vi "tkrsa6100 Status Regs.vi"(0 "VISA Resource Name":refnum<visa-resource-name>, 5 "Set/Read\nStatus Register (SET)":enum16{"SET", "READ"}(ring), 7 "Register (PRESET)":T1(ring), 9 "Register # (0)":i32 max=32767 step=1, 11 "error in (no error)":errorcluster {"code" format="%#.0f"}) -> (4 "dup VISA Resource Name":refnum<visa-resource-name>, 6 "Register #\nResponse String":string, 8 "Register Bits Array":bool[](array[boolean]), 10 "Register #":i32, 15 "error out":errorcluster {"code" format="%#.0f"})   [LabVIEW 2020, in "Library Instrument & Equipement.lvlib" / "Library Spectrum Analyser.lvlib"]
doc: "Prerequisites for use:\n\nNone. This VI is valid in all measurement views.\n\nThis VI sets or reads the current instrument status registers. To use the VI pass either SET or READ to enumerated control Set/Read Acquisition Setting(SET), pass the input register to be written or read to enumerated control Register(PRESET), and if writing a register, pass the number to numeric control Register # (0). Functions that are write-only are followed by (SET), functions that are read-only are followed by (READ). \n\nFirst error in (no error) is checked by tkrsa6100 Write/Read WError Query.vi for any pending errors.\n\nIf error in status is ERROR:\n\nerror in (no error) and VISA Resource Name are passed straight through to error out and dup VISA Resource Name of the tkrsa6100 Write/Read WError Query.vi and returned to the calling function. No commands are processed.\n\nIf error in status is NO ERROR:\n\nThe register settings are set or read per the values passed to controls Register(PRESET) and Register #(0).\n\nIf SET is passed the following registers can be written per the value passed to numeric control Register # (0): \n\nPRESET (SET). This presets the registers to their default settings. No other parameters are necessary to be passed.\n\nThe following are the registers that can be written:\n\nOPERATION:ENABLE\nOPERATION:PTRANSITION\nOPERATION:NTRANSITION\nQUESTIONABLE:ENABLE\nQUESTIONABLE:PTRANSITION\nQUESTIONABLE:NTRANSITION\nQUESTIONABLE:FREQUENCY:ENABLE\nQUESTIONABLE: FREQUENCY:PTRANSITION\nQUESTIONABLE: FREQUENCY:NTRANSITION\n*QUESTIONABLE:INTEGRITY:ENABLE\n*QUESTIONABLE: INTEGRITY:PTRANSITION\n*QUESTIONABLE: INTEGRITY:NTRANSITION\nQUESTIONABLE:CALIBRATION:ENABLE\nQUESTIONABLE: CALIBRATION:PTRANSITION\nQUESTIONABLE: CALIBRATION:NTRANSITION\n*QUESTIONABLE:POWER:ENABLE\n*QUESTIONABLE: POWER:PTRANSITION\n*QUESTIONABLE: POWER:NTRANSITION\n*QUESTIONABLE:TEMPERATURE:ENABLE\n*QUESTIONABLE: TEMPERATURE:PTRANSITION\n*QUESTIONABLE: TEMPERATURE:NTRANSITION\n\n*These registers currently have no bits assigned in them but are included for completeness.\n\nValues 0 to 32767 can be written to the registers\n.\nWrite a 1 to the bit of interest in the ENABLE registers to enable them.\n\nIf a 1 is written to the bit of interest in the PTRANSITION register the bit will be set in the EVENT register if a low to high transition is detected.\n\nIf a 1 is written to the bit of interest in the NTRANSITION register the bit will be set in the EVENT register if a high to low transition is detected.\n\nIf a 1 is written to the bit of interest in both the PTRANSITION and NTRANSITION registers the bit will be set in the EVENT register if any transition is detected.\n\nRefer to Section 3 (Status and Events) of the Programmer's Manual for assigned register bits and further information.\n\nAfter the correct command string is selected it is passed to tkrsa6100 Write/Read wError Query.vi.\n\nIf READ is passed the following registers can be read.\n\nOPERATION:CONDITION\nOPERATION:ENABLE\nOPERATION:EVENT\nOPERATION:PTRANSITION\nOPERATION:NTRANSITION\nQUESTIONABLE:CONDITION\nQUESTIONABLE:ENABLE\nQUESTIONABLE:EVENT\nQUESTIONABLE:PTRANSITION\nQUESTIONABLE:NTRANSITION\nQUESTIONABLE: FREQUENCY:CONDITION\nQUESTIONABLE:FREQUENCY:ENABLE\nQUESTIONABLE: FREQUENCY:EVENT\nQUESTIONABLE: FREQUENCY:PTRANSITION\nQUESTIONABLE: FREQUENCY:NTRANSITION\n*QUESTIONABLE:INTEGRITY:CONDITION\n\n*QUESTIONABLE:INTEGRITY:ENABLE\n*QUESTIONABLE:INTEGRITY:EVENT\n*QUESTIONABLE: INTEGRITY:PTRANSITION\n*QUESTIONABLE: INTEGRITY:NTRANSITION\nQUESTIONABLE:CALIBRATION:CONDITION\nQUESTIONABLE:CALIBRATION:ENABLE\nQUESTIONABLE:CALIBRATION:EVENT\nQUESTIONABLE: CALIBRATION:PTRANSITION\nQUESTIONABLE: CALIBRATION:NTRANSITION\n*QUESTIONABLE:POWER:CONDITION\n*QUESTIONABLE:POWER:ENABLE\n*QUESTIONABLE:POWER:EVENT\n*QUESTIONABLE: POWER:PTRANSITION\n*QUESTIONABLE: POWER:NTRANSITION\n*QUESTIONABLE:TEMPERATURE:CONDITION\n*QUESTIONABLE:TEMPERATURE:ENABLE\n*QUESTIONABLE:TEMPERATURE:EVENT\n*QUESTIONABLE: TEMPERATURE:PTRANSITION\n*QUESTIONABLE: TEMPERATURE:NTRANSITION\n\n*These registers currently have no bits assigned in them but are included for completeness.\n\nReturn values are 0 to 32767. The returned numeric value is also converted to a 16 bit boolean array Error Bits Array for a visual indication of active bits.\n\nThe appropriate command/query string is passed to tkrsa6100 Write/Read wError Query.vi. VI Input Error Query? is set to YES by default so query SYST:ERR? is appended to the command string and any current error information is displayed in cluster Error Out.\nOn completion dup VISA Resource Name, Error Out, and Measurement Response String are returned to the calling function."
uses:
  Library Spectrum Analyser.lvlib
panel:
  # "RSA6100 Status Register Driver"
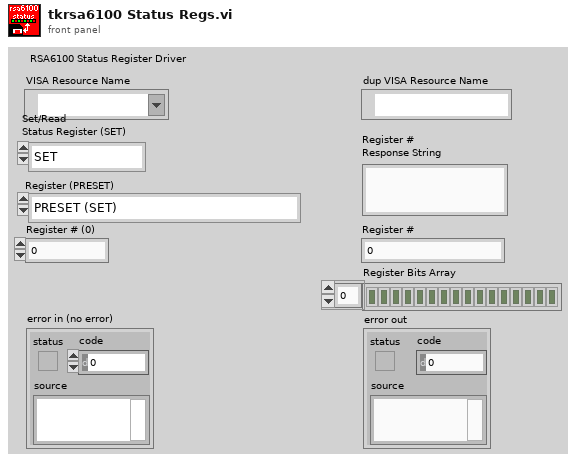
[diagram p1: front panel]
types:
  T1 = enum16{"PRESET (SET)", "OPERATION CONDITION (READ)", "OPERATION ENABLE", "OPERATION EVENT (READ)", "OPERATION PTRANSITION", "OPERATION NTRANSITION", "QUESTIONABLE CONDITION (READ)", "QUESTIONABLE ENABLE", "QUESTIONABLE EVENT (READ)", "QUESTIONABLE PTRANSITION", "QUESTIONABLE NTRANSITION", "QUESTIONABLE FREQ CONDITION (READ)", "QUESTIONABLE FREQ ENABLE", "QUESTIONABLE FREQ EVENT (READ)", "QUESTIONABLE FREQ PTRANSITION", "QUESTIONABLE FREQ NTRANSITION", "QUESTIONABLE INTEGRITY CONDITION (READ)", "QUESTIONABLE INTEGRITY ENABLE", "QUESTIONABLE INTEGRITY EVENT (READ)", "QUESTIONABLE INTEGRITY PTRANSITION", "QUESTIONABLE INTEGRITY NTRANSITION", "QUESTIONABLE CALIB CONDITION (READ)", "QUESTIONABLE CALIB ENABLE", "QUESTIONABLE CALIB EVENT (READ)", "QUESTIONABLE CALIB PTRANSITON", "QUESTIONABLE CALIB NTRANSITION", "QUESTIONABLE POWER CONDITION (READ)", "QUESTIONABLE POWER ENABLE", "QUESTIONABLE POWER EVENT (READ)", "QUESTIONABLE POWER PTRANSITION", "QUESTIONABLE POWER NTRANSITION", "QUESTIONABLE TEMP CONDITION (READ)", "QUESTIONABLE TEMP ENABLE", "QUESTIONABLE TEMP EVENT (READ)", "QUESTIONABLE TEMP PTRANSITION", "QUESTIONABLE TEMP NTRANSITION"}
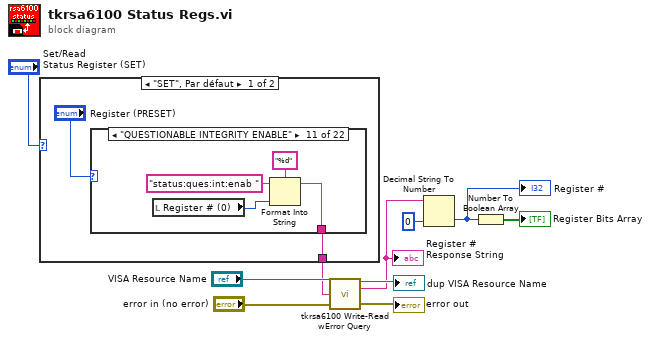
[diagram p0: block diagram]
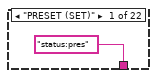
[diagram p2: hidden frame]
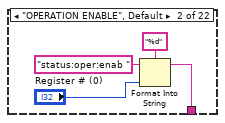
[diagram p3: hidden frame]
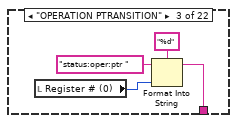
[diagram p4: hidden frame]
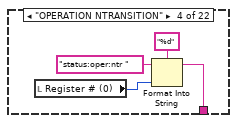
[diagram p5: hidden frame]
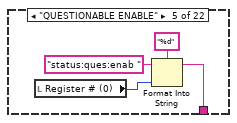
[diagram p6: hidden frame]
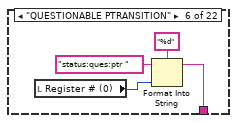
[diagram p7: hidden frame]
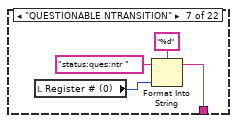
[diagram p8: hidden frame]
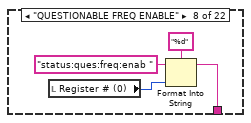
[diagram p9: hidden frame]
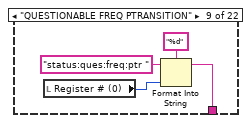
[diagram p10: hidden frame]
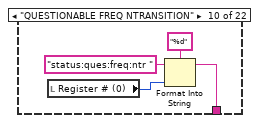
[diagram p11: hidden frame]
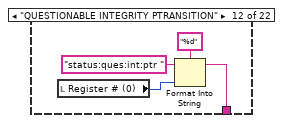
[diagram p12: hidden frame]
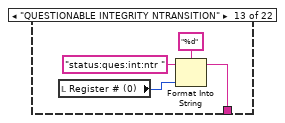
[diagram p13: hidden frame]
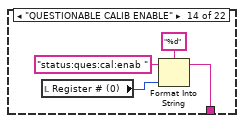
[diagram p14: hidden frame]
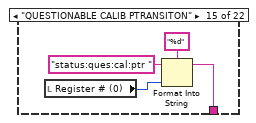
[diagram p15: hidden frame]
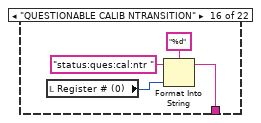
[diagram p16: hidden frame]
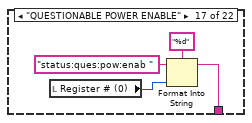
[diagram p17: hidden frame]
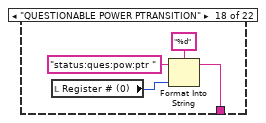
[diagram p18: hidden frame]
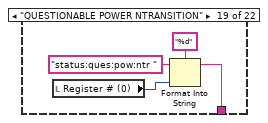
[diagram p19: hidden frame]
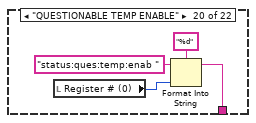
[diagram p20: hidden frame]
diagram:
  n1 = case shown="\"SET\", Par défaut" "Set/Read\nStatus Register (SET)" {
    tunnel: [w12 w98] -> w5
    frame "SET", Default {
      n2 = case shown="\"QUESTIONABLE INTEGRITY ENABLE\"" "Register (PRESET)" {
        tunnel: ["status:pres" ("initial string") w14 w19 w23 w27 w31 w35 w39 w43 w47 w51 w55 w59 w63 w67 w71 w75 w79 w83 w87 w91 w95] -> w12
        frame "PRESET (SET)" {
        }
        frame "OPERATION ENABLE", Default {
          n3 = Format Into String(format string="%d", initial string="status:oper:enab ", "Register # (0)") -> (resulting string=w14:string)  [unwired: 1 in, 1 out]
        }
        frame "OPERATION PTRANSITION" {
          n4 = local read "Register # (0)"() -> (w18:i32)
          n5 = Format Into String(format string="%d", initial string="status:oper:ptr ", w18) -> (resulting string=w19:string)  [unwired: 1 in, 1 out]
        }
        frame "OPERATION NTRANSITION" {
          n6 = local read "Register # (0)"() -> (w22:i32)
          n7 = Format Into String(format string="%d", initial string="status:oper:ntr ", w22) -> (resulting string=w23:string)  [unwired: 1 in, 1 out]
        }
        frame "QUESTIONABLE ENABLE" {
          n8 = local read "Register # (0)"() -> (w26:i32)
          n9 = Format Into String(format string="%d", initial string="status:ques:enab ", w26) -> (resulting string=w27:string)  [unwired: 1 in, 1 out]
        }
        frame "QUESTIONABLE PTRANSITION" {
          n10 = local read "Register # (0)"() -> (w30:i32)
          n11 = Format Into String(format string="%d", initial string="status:ques:ptr ", w30) -> (resulting string=w31:string)  [unwired: 1 in, 1 out]
        }
        frame "QUESTIONABLE NTRANSITION" {
          n12 = local read "Register # (0)"() -> (w34:i32)
          n13 = Format Into String(format string="%d", initial string="status:ques:ntr ", w34) -> (resulting string=w35:string)  [unwired: 1 in, 1 out]
        }
        frame "QUESTIONABLE FREQ ENABLE" {
          n14 = local read "Register # (0)"() -> (w38:i32)
          n15 = Format Into String(format string="%d", initial string="status:ques:freq:enab ", w38) -> (resulting string=w39:string)  [unwired: 1 in, 1 out]
        }
        frame "QUESTIONABLE FREQ PTRANSITION" {
          n16 = local read "Register # (0)"() -> (w42:i32)
          n17 = Format Into String(format string="%d", initial string="status:ques:freq:ptr ", w42) -> (resulting string=w43:string)  [unwired: 1 in, 1 out]
        }
        frame "QUESTIONABLE FREQ NTRANSITION" {
          n18 = local read "Register # (0)"() -> (w46:i32)
          n19 = Format Into String(format string="%d", initial string="status:ques:freq:ntr ", w46) -> (resulting string=w47:string)  [unwired: 1 in, 1 out]
        }
        frame "QUESTIONABLE INTEGRITY ENABLE" {
          n20 = local read "Register # (0)"() -> (w50:i32)
          n21 = Format Into String(format string="%d", initial string="status:ques:int:enab ", w50) -> (resulting string=w51:string)  [unwired: 1 in, 1 out]
        }
        frame "QUESTIONABLE INTEGRITY PTRANSITION" {
          n22 = local read "Register # (0)"() -> (w54:i32)
          n23 = Format Into String(format string="%d", initial string="status:ques:int:ptr ", w54) -> (resulting string=w55:string)  [unwired: 1 in, 1 out]
        }
        frame "QUESTIONABLE INTEGRITY NTRANSITION" {
          n24 = local read "Register # (0)"() -> (w58:i32)
          n25 = Format Into String(format string="%d", initial string="status:ques:int:ntr ", w58) -> (resulting string=w59:string)  [unwired: 1 in, 1 out]
        }
        frame "QUESTIONABLE CALIB ENABLE" {
          n26 = local read "Register # (0)"() -> (w62:i32)
          n27 = Format Into String(format string="%d", initial string="status:ques:cal:enab ", w62) -> (resulting string=w63:string)  [unwired: 1 in, 1 out]
        }
        frame "QUESTIONABLE CALIB PTRANSITON" {
          n28 = local read "Register # (0)"() -> (w66:i32)
          n29 = Format Into String(format string="%d", initial string="status:ques:cal:ptr ", w66) -> (resulting string=w67:string)  [unwired: 1 in, 1 out]
        }
        frame "QUESTIONABLE CALIB NTRANSITION" {
          n30 = local read "Register # (0)"() -> (w70:i32)
          n31 = Format Into String(format string="%d", initial string="status:ques:cal:ntr ", w70) -> (resulting string=w71:string)  [unwired: 1 in, 1 out]
        }
        frame "QUESTIONABLE POWER ENABLE" {
          n32 = local read "Register # (0)"() -> (w74:i32)
          n33 = Format Into String(format string="%d", initial string="status:ques:pow:enab ", w74) -> (resulting string=w75:string)  [unwired: 1 in, 1 out]
        }
        frame "QUESTIONABLE POWER PTRANSITION" {
          n34 = local read "Register # (0)"() -> (w78:i32)
          n35 = Format Into String(format string="%d", initial string="status:ques:pow:ptr ", w78) -> (resulting string=w79:string)  [unwired: 1 in, 1 out]
        }
        frame "QUESTIONABLE POWER NTRANSITION" {
          n36 = local read "Register # (0)"() -> (w82:i32)
          n37 = Format Into String(format string="%d", initial string="status:ques:pow:ntr ", w82) -> (resulting string=w83:string)  [unwired: 1 in, 1 out]
        }
        frame "QUESTIONABLE TEMP ENABLE" {
          n38 = local read "Register # (0)"() -> (w86:i32)
          n39 = Format Into String(format string="%d", initial string="status:ques:temp:enab ", w86) -> (resulting string=w87:string)  [unwired: 1 in, 1 out]
        }
        frame "QUESTIONABLE TEMP PTRANSITION" {
          n40 = local read "Register # (0)"() -> (w90:i32)
          n41 = Format Into String(format string="%d", initial string="status:ques:temp:ptr ", w90) -> (resulting string=w91:string)  [unwired: 1 in, 1 out]
        }
        frame "QUESTIONABLE TEMP NTRANSITION" {
          n42 = local read "Register # (0)"() -> (w94:i32)
          n43 = Format Into String(format string="%d", initial string="status:ques:temp:ntr ", w94) -> (resulting string=w95:string)  [unwired: 1 in, 1 out]
        }
      }
    }
    frame "READ" {
      n44 = local read "Register (PRESET)"() -> (w99:T1)
      n45 = case shown="\"OPERATION CONDITION (READ)\", Par défaut" w99 {
        tunnel: ["status:oper:cond?" "status:oper:enab?" "status:oper:even?" "status:oper:ptr?" "status:oper:ntr?" "status:ques:cond?" "status:ques:enab?" "status:ques:even?" "status:ques:ptr?" "status:ques:ntr?" "status:ques:freq:cond?" "status:ques:freq:enab?" "status:ques:freq:even?" "status:ques:freq:ptr?" "status:ques:freq:ntr?" "status:ques:int:cond?" "status:ques:int:enab?" "status:ques:int:even?" "status:ques:int:ptr?" "status:ques:int:ntr?" "status:ques:cal:cond?" "status:ques:cal:enab?" "status:ques:cal:even?" "status:ques:cal:ptr?" "status:ques:cal:ntr?" "status:ques:pow:cond?" "status:ques:pow:enab?" "status:ques:pow:even?" "status:ques:pow:ptr?" "status:ques:pow:ntr?" "status:ques:temp:cond?" "status:ques:temp:enab?" "status:ques:temp:even?" "status:ques:temp:ptr?" "status:ques:temp:ntr?"] -> w98
        frame "OPERATION CONDITION (READ)", Default {
        }
        frame "OPERATION ENABLE" {
        }
        frame "OPERATION EVENT (READ)" {
        }
        frame "OPERATION PTRANSITION" {
        }
        frame "OPERATION NTRANSITION" {
        }
        frame "QUESTIONABLE CONDITION (READ)" {
        }
        frame "QUESTIONABLE ENABLE" {
        }
        frame "QUESTIONABLE EVENT (READ)" {
        }
        frame "QUESTIONABLE PTRANSITION" {
        }
        frame "QUESTIONABLE NTRANSITION" {
        }
        frame "QUESTIONABLE FREQ CONDITION (READ)" {
        }
        frame "QUESTIONABLE FREQ ENABLE" {
        }
        frame "QUESTIONABLE FREQ EVENT (READ)" {
        }
        frame "QUESTIONABLE FREQ PTRANSITION" {
        }
        frame "QUESTIONABLE FREQ NTRANSITION" {
        }
        frame "QUESTIONABLE INTEGRITY CONDITION (READ)" {
        }
        frame "QUESTIONABLE INTEGRITY ENABLE" {
        }
        frame "QUESTIONABLE INTEGRITY EVENT (READ)" {
        }
        frame "QUESTIONABLE INTEGRITY PTRANSITION" {
        }
        frame "QUESTIONABLE INTEGRITY NTRANSITION" {
        }
        frame "QUESTIONABLE CALIB CONDITION (READ)" {
        }
        frame "QUESTIONABLE CALIB ENABLE" {
        }
        frame "QUESTIONABLE CALIB EVENT (READ)" {
        }
        frame "QUESTIONABLE CALIB PTRANSITON" {
        }
        frame "QUESTIONABLE CALIB NTRANSITION" {
        }
        frame "QUESTIONABLE POWER CONDITION (READ)" {
        }
        frame "QUESTIONABLE POWER ENABLE" {
        }
        frame "QUESTIONABLE POWER EVENT (READ)" {
        }
        frame "QUESTIONABLE POWER PTRANSITION" {
        }
        frame "QUESTIONABLE POWER NTRANSITION" {
        }
        frame "QUESTIONABLE TEMP CONDITION (READ)" {
        }
        frame "QUESTIONABLE TEMP ENABLE" {
        }
        frame "QUESTIONABLE TEMP EVENT (READ)" {
        }
        frame "QUESTIONABLE TEMP PTRANSITION" {
        }
        frame "QUESTIONABLE TEMP NTRANSITION" {
        }
      }
    }
  }
  n46 = call "tkrsa6100 Write-Read wError Query.vi"("VISA Resource Name"="VISA Resource Name", "Command (Empty String)"=w5, "error in (no error)"="error in (no error)") -> ("dup VISA Resource Name"=→"dup VISA Resource Name":refnum<visa-resource-name>, "Response"=w4:string, "error out"=→"error out":errorcluster)  [unwired: 4 in, 6 out]
  "Register #\nResponse String" <- w4
  n47 = Decimal String To Number(string=w4, default (0L)=u16 0 ("default (0 I32)")) -> (number=w1:u16)  [unwired: 2 out]
  "Register #" <- w1
  n48 = Number To Boolean Array(number=w1) -> (Boolean array=→"Register Bits Array":bool[])
